vi "C1--end cube.vi"(8 "Command Info In":T1, 10 "C1--end cube":T4={"1a"=0.0, "2d"=0.0, "2s"=0.0, "3g"=0.65, "4t"=1.0}, 11 "Switch":string) -> (0 "Command Info Out":T1)   [LabVIEW 2017]
uses:
  Block Clusters/C1--end cube.ctl
  <vilib>/Rock Robotics/WPI/Framework/Command Status Info.ctl
  <vilib>/Rock Robotics/WPI/Framework/Completion Status.ctl
  <vilib>/Rock Robotics/WPI/Framework/Completion Notifier.ctl
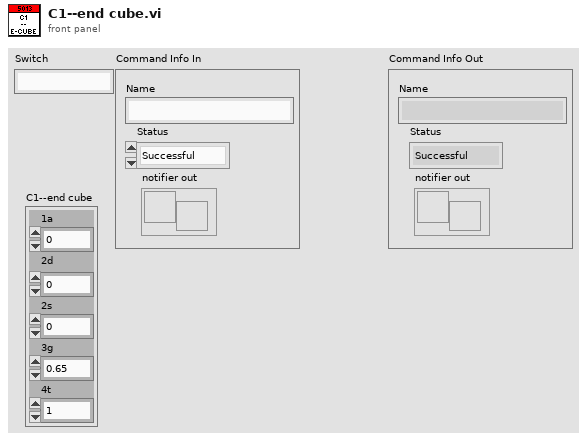
[diagram p1: front panel]
types:
  T1 = typedef "Command Status Info.ctl" = cluster{"Name":string, "Status":T2, "notifier out":T3}
  T2 = typedef "Completion Status.ctl" = enum16{"Successful", "Aborted", "Incomplete"}
  T3 = typedef "Completion Notifier.ctl" = refnum<notifier>
  T4 = typedef "C1--end cube.ctl" = cluster{"1a":dbl, "2d":dbl, "2s":dbl, "3g":dbl, "4t":dbl}
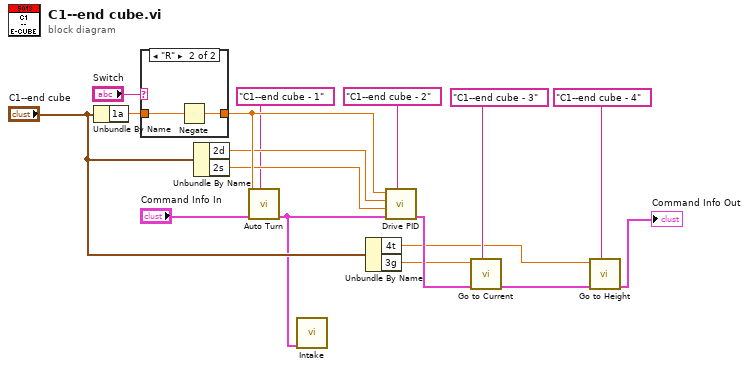
[diagram p0: block diagram]
diagram:
  n1 = Unbundle By Name("C1--end cube") -> ("1a"=w17:dbl)
  n2 = case shown="\"R\"" "Switch" {
    tunnel: w17 -> [w18 w20]
    tunnel: [w18 w19] -> w16
    frame "L", Default {
    }
    frame "R" {
      n3 = Negate(x=w20) -> (-x=w19:dbl)
    }
  }
  n4 = Unbundle By Name("C1--end cube") -> ("2d"=w15:dbl, "2s"=w14:dbl)
  n5 = call "Auto Turn.vi"("Description"="C1--end cube - 1", "Command Info In"="Command Info In", "Target Angle"=w16) -> ("Command Info Out"=w5:T1)  [unwired: 8 in]
  n6 = call "Intake.vi"("Command Info In"=w5) -> ()  [unwired: 10 in, 1 out]
  n7 = Unbundle By Name("C1--end cube") -> ("4t"=w3:dbl, "3g"=w7:dbl)
  n8 = call "Drive PID.vi"("Description"="C1--end cube - 2", "Command Info In"=w5, "Speed"=w14, "Distance"=w15, "Target Angle"=w16) -> ("Command Info Out"=w9:T1)  [unwired: 6 in]
  n9 = call "Go to Current.vi"("Description"="C1--end cube - 3", "Command Info In"=w9, "Setpoint"=w7) -> ("Command Info Out"=w4:T1)  [unwired: 8 in]
  n10 = call "Go to Height.vi"("Description"="C1--end cube - 4", "Command Info In"=w4, "Target Height (in)"=w3) -> ("Command Info Out"=→"Command Info Out":T1)  [unwired: 8 in]
